vi "Permutation.vi"() -> ()   [LabVIEW 2015]
panel:
  out "nPr":i32
  out "nCr":i32
  in  "R":i32
  in  "N":i32
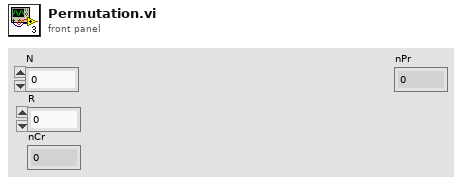
[diagram p1: front panel]
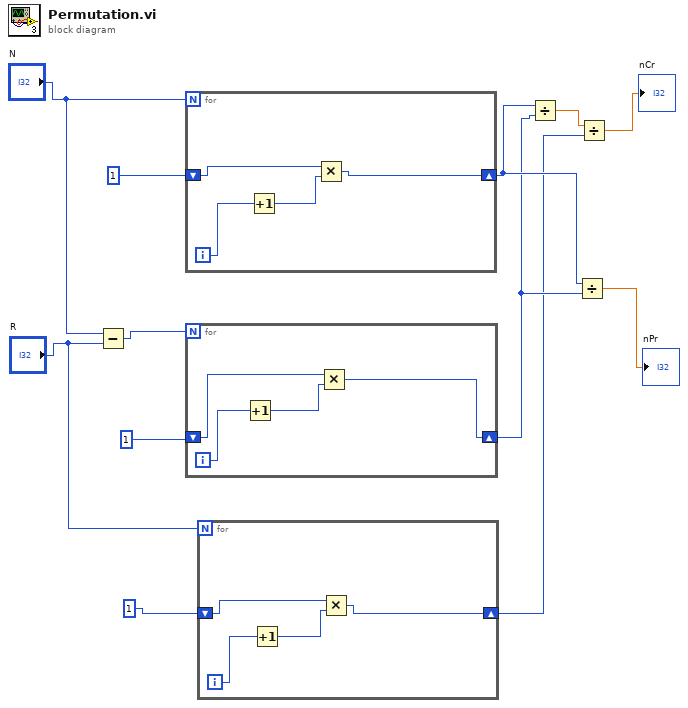
[diagram p0: block diagram]
diagram:
  n1 = Subtract(x="N", y="R") -> (x-y=w10:i32)
  n2 = for {
    N: "N" -> [_]
    shift-right: [w13] -> w6
    shift-left: 1 -> [w14]
    i -> [w16]
    n3 = Increment(x=w16) -> (x+1=w15:i32)
    n4 = Multiply(x=w14, y=w15) -> (x*y=w13:i32)
  }
  n5 = for {
    N: w10 -> [_]
    shift-right: [w17] -> w5
    shift-left: 1 -> [w19]
    i -> [w20]
    n6 = Increment(x=w20) -> (x+1=w18:i32)
    n7 = Multiply(x=w19, y=w18) -> (x*y=w17:i32)
  }
  n8 = for {
    N: "R" -> [_]
    shift-right: [w21] -> w3
    shift-left: 1 -> [w23]
    i -> [w24]
    n9 = Increment(x=w24) -> (x+1=w22:i32)
    n10 = Multiply(x=w23, y=w22) -> (x*y=w21:i32)
  }
  n11 = Divide(x=w6, y=w5) -> (x/y=w4:dbl)
  n12 = Divide(x=w6, y=w5) -> (x/y=→"nPr":dbl)
  n13 = Divide(x=w4, y=w3) -> (x/y=→"nCr":dbl)
